vi "Command URL Test.vi"() -> ()   [LabVIEW 2019]
panel:
  in  "Parameter Values":string[](array[string])=["Ok", "TRUE", "23467", "FALSE", "value"]
  in  "Parameter Keys":string[](array[string])=["param_1", "param_2_test", "param_three", "my_custom_param", "test"]
  in  "Scanner IP Address":string="10.48.0.57"
  in  "Command String":string="my_command"
  out "Command URL out":string="http://10.48.0.57/cmd/my_command?param_1=Ok&param_2_test=TRUE&param_three=23467&my_custom_param=FALSE&test=value"
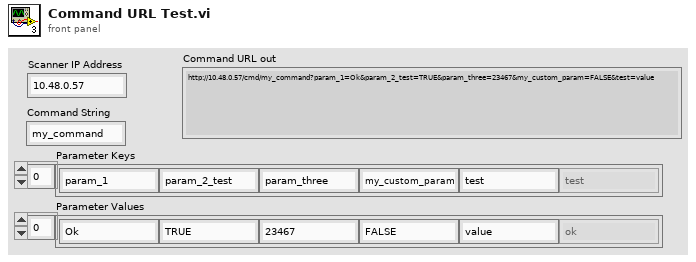
[diagram p1: front panel]
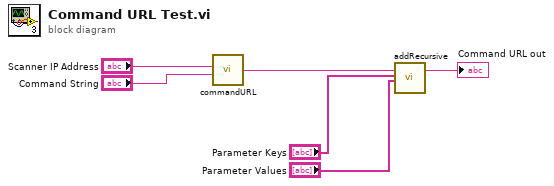
[diagram p0: block diagram]
diagram:
  n1 = call "commandURL.vi"("Command String"="Command String", "Scanner IP Address"="Scanner IP Address") -> ("Command URL"=w3:string)  [unwired: 4 in]
  n2 = call "addRecursive.vi"("Command URL in"=w3, "Parameter Key"="Parameter Keys", "Parameter Value"="Parameter Values") -> ("Command URL out"=→"Command URL out":string)  [unwired: 13 in, 3 out]
